vi "valve_control.vi"(2 "Loop Time [ms]":u32, 3 "PID Control":T1={"proportional gain (Kc)"=1.0, "integral time (Ti, min)"=0.01, "derivative time (Td, min)"=0.0, "Valve Voltage [V]"=0.0, "Min % Open"=2.0, "Max % Open"=3.0, "Reinitialize?"=FALSE, "Valve On/Off"=FALSE, "Mode"=FALSE, "Full Flow Rate"=0.0, "Flow Set Point [g/s]"=0.0, "AutoTune"=FALSE, "Flow"={"Flow rate [g/s]"=0.0, "Line Density [g/cm^3]"=0.0}} {"Flow Set Point [g/s]" format="%.2f"; "Full Flow Rate" format="%.2f"; "Max % Open" min=0.0 max=100.0 format="%.2f"; "Min % Open" min=0.0 max=100.0 format="%.2f"; "Valve Voltage [V]" min=1.0 max=5.0 step=0.01 format="%.4f"; "derivative time (Td, min)" format="%.3f"; "integral time (Ti, min)" format="%.3f"; "proportional gain (Kc)" format="%.3f"}) -> (0 "Valve Voltage [V]":dbl, 1 "PID Control Output":T1={"proportional gain (Kc)"=1.0, "integral time (Ti, min)"=0.01, "derivative time (Td, min)"=0.0, "Valve Voltage [V]"=0.0, "Min % Open"=2.0, "Max % Open"=3.0, "Reinitialize?"=FALSE, "Valve On/Off"=FALSE, "Mode"=FALSE, "Full Flow Rate"=0.0, "Flow Set Point [g/s]"=0.0, "AutoTune"=FALSE, "Flow"={"Flow rate [g/s]"=0.0, "Line Density [g/cm^3]"=0.0}} {"Flow Set Point [g/s]" format="%.2f"; "Full Flow Rate" format="%.2f"; "Max % Open" min=0.0 max=100.0 format="%.2f"; "Min % Open" min=0.0 max=100.0 format="%.2f"; "Valve Voltage [V]" min=1.0 max=5.0 step=0.01 format="%.4f"; "derivative time (Td, min)" format="%.3f"; "integral time (Ti, min)" format="%.3f"; "proportional gain (Kc)" format="%.3f"})   [LabVIEW 2017]
uses:
  valve_pid_control.ctl
  <vilib>/addons/control/pid/NI_PID_autopid.lvlib
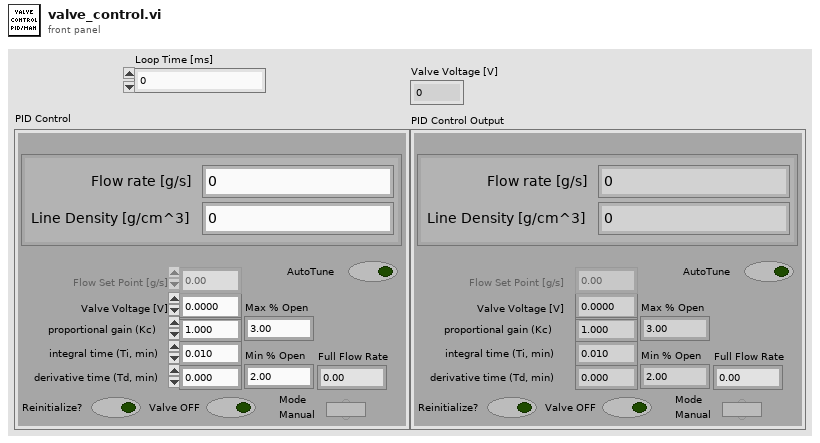
[diagram p1: front panel]
types:
  T1 = typedef "valve_pid_control.ctl" = cluster{"proportional gain (Kc)":dbl, "integral time (Ti, min)":dbl, "derivative time (Td, min)":dbl, "Valve Voltage [V]":dbl, "Min % Open":dbl, "Max % Open":dbl, "Reinitialize?":bool, "Valve On/Off":bool, "Mode":bool, "Full Flow Rate":dbl, "Flow Set Point [g/s]":dbl, "AutoTune":bool, "Flow":cluster{"Flow rate [g/s]":dbl, "Line Density [g/cm^3]":dbl}}
  T2 = cluster{"proportional gain (Kc)":dbl, "integral time (Ti, min)":dbl, "derivative time (Td, min)":dbl}
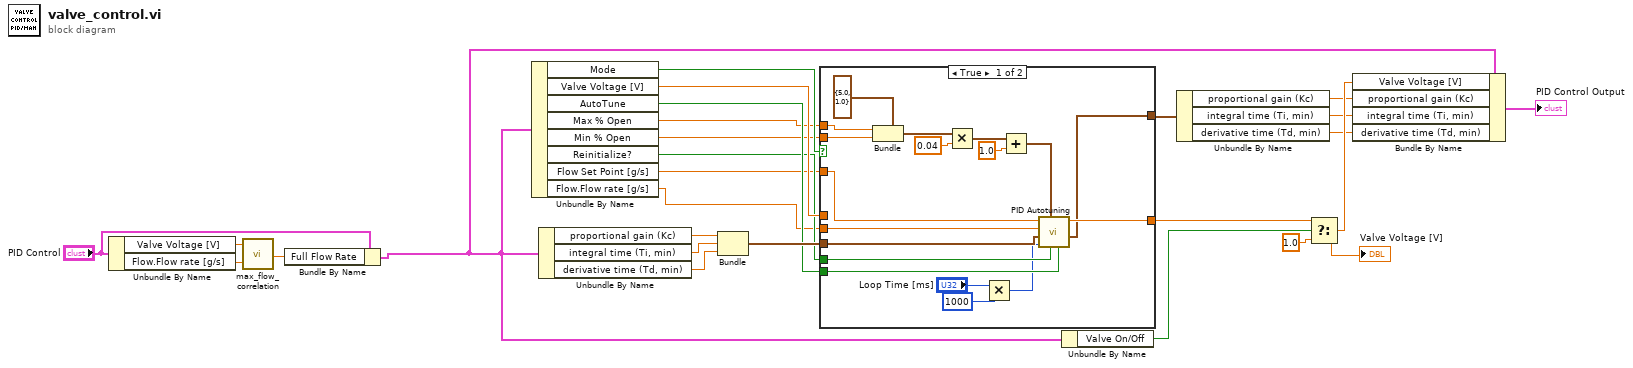
[diagram p0: block diagram]
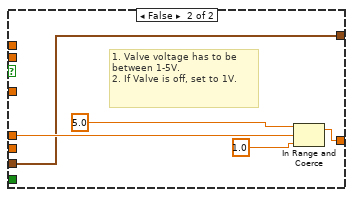
[diagram p2: hidden frame]
diagram:
  n1 = Unbundle By Name("PID Control") -> ("Valve Voltage [V]"=w6:dbl, "Flow.Flow rate [g/s]"=w5:dbl)
  n2 = call "max_flow_correlation.vi"("Current Flow Rate"=w5, "Current Voltage"=w6) -> ("Max Flow Rate"=w3:dbl)
  n3 = Bundle By Name(cluster="PID Control", "Full Flow Rate"=w3) -> (w2:T1)
  n4 = Unbundle By Name(w2) -> ("Mode"=w26:bool, "Valve Voltage [V]"=w23:dbl, "AutoTune"=w24:bool, "Max % Open"=w18:dbl, "Min % Open"=w17:dbl, "Reinitialize?"=w22:bool, "Flow Set Point [g/s]"=w11:dbl, "Flow.Flow rate [g/s]"=w1:dbl)
  n5 = Unbundle By Name(w2) -> ("proportional gain (Kc)"=w21:dbl, "integral time (Ti, min)"=w20:dbl, "derivative time (Td, min)"=w19:dbl)
  n6 = Bundle("proportional gain (Kc)"=w21, "integral time (Ti, min)"=w20, "derivative time (Td, min)"=w19) -> (w25:T2)  [unwired: 1 in]
  n7 = case shown="True" w26 {
    tunnel: [w39 w46] -> w14
    tunnel: w23 -> [_ w47]
    tunnel: w1 -> [w44 _]
    tunnel: w25 -> [w43 w45]
    tunnel: w22 -> [w42 _]
    tunnel: w18 -> [w41 _]
    tunnel: w17 -> [w40 _]
    tunnel: w24 -> [w38 _]
    tunnel: w11 -> [w33 _]
    tunnel: [w27 w45] -> w10
    frame True {
      n8 = Bundle(cluster=cluster{"output high":dbl, "output low":dbl} {"output high"=5.0, "output low"=1.0} ("output range"), "output high"=w41, "output low"=w40) -> (w35:cluster{"output high":dbl, "output low":dbl})
      n9 = Multiply(x=w35, y=0.04) -> (x*y=w36:cluster{"output high":dbl, "output low":dbl})
      n10 = Multiply(x="Loop Time [ms]", y=u32 1000) -> (x*y=w28:u32)
      n11 = Add(x=w36, y=1.0) -> (x+y=w32:cluster{"output high":dbl, "output low":dbl})
      n12 = call <vilib>:"PID Autotuning.vi"("autotune? (F)"=w38, "reinitialize? (F)"=w42, "output range"=w32, "dt (s)"=w28, "PID gains"=w43, "process variable"=w44, "setpoint"=w33) -> ("PID gains out"=w27:T2, "output"=w39:dbl)  [unwired: 1 in, 2 out]
    }
    frame False {
      # "1. Valve voltage has to be between 1-5V.\n2. If Valve is off, set to 1V."
      n13 = In Range and Coerce(upper limit=5.0, x=w47, lower limit=1.0) -> (coerced(x)=w46:dbl)  [unwired: 1 out]
    }
  }
  n14 = Unbundle By Name(w2) -> ("Valve On/Off"=w13:bool)
  n15 = Unbundle By Name(w10) -> ("proportional gain (Kc)"=w9:dbl, "integral time (Ti, min)"=w8:dbl, "derivative time (Td, min)"=w7:dbl)
  n16 = Select(t=w14, s=w13, f=1.0) -> (s? t:f=w12:dbl)
  "Valve Voltage [V]" <- w12
  n17 = Bundle By Name(cluster=w2, "Valve Voltage [V]"=w12, "proportional gain (Kc)"=w9, "integral time (Ti, min)"=w8, "derivative time (Td, min)"=w7) -> (→"PID Control Output":T1)
